vi "Version_4.9_8_on-chip_valves_for25ulSyringe_withModfied_Plunging.vi"() -> ()   [LabVIEW 2020] (continued)
                                n4611 = local read "VISA Refnum in\nfor Pump"() -> (w5031:refnum<visa-resource-name>)
                                n4612 = local read "Initial Plunger Position"() -> (w5030:dbl)
                                n4613 = local read "Volume of Syringe"() -> (w5028:dbl)
                                n4614 = while {
                                tunnel: w5030 -> [w5038]
                                tunnel: w5031 -> [w5037]
                                tunnel: w5029 -> [w5036]
                                tunnel: w5028 -> [w5035]
                                stop <- w5033 stop-if-true
                                n4615 = stacked-sequence {
                                tunnel: w5038 -> [w5045 _]
                                tunnel: w5037 -> [w5044 w5065]
                                tunnel: w5036 -> [w5043 _]
                                tunnel: w5035 -> [w5042 _]
                                tunnel: [_ w5063] -> w5033
                                frame #0 {
                                n4616 = call "AbsolutePlungerPosition (SubVI).vi"("VISA Refnum in"=w5044) -> ("Plunger Position"=w5041:i32)  [unwired: 10 in]
                                n4617 = case shown="\"Standard Pumping\", Default" w5043 {
                                tunnel: w5045 -> [w5050 w5059]
                                tunnel: w5041 -> [w5051 w5058]
                                tunnel: [w5049 w5056] -> w5040
                                tunnel: w5042 -> [w5048 w5057]
                                frame "Standard Pumping", Default {
                                n4618 = Subtract(x=w5050, y=w5051) -> (x-y=w5047:dbl)
                                n4619 = Absolute Value(x=w5047) -> (abs(x)=w5046:dbl)
                                n4620 = Multiply(x=w5046, y=w5048) -> (x*y=w5053:dbl)
                                n4621 = Divide(x=w5053, y=3000.0) -> (x/y=w5049:dbl)
                                }
                                frame "High Resolution Pumping" {
                                n4622 = Subtract(x=w5059, y=w5058) -> (x-y=w5055:dbl)
                                n4623 = Absolute Value(x=w5055) -> (abs(x)=w5054:dbl)
                                n4624 = Multiply(x=w5054, y=w5057) -> (x*y=w5061:dbl)
                                n4625 = Divide(x=w5061, y=24000.0) -> (x/y=w5056:dbl)
                                }
                                }
                                n4626 = local write "Volume being Injected \nin this process"(w5040) -> ()
                                }
                                frame #1 {
                                n4627 = local read "Stopper that ends \nthe main loops"() -> (w5062:bool)
                                n4628 = call "LSPOneStatus (SubVI).vi"("VISA Refnum in"=w5065) -> ("read buffer"=w5067:string)  [unwired: 10 in]
                                n4629 = call <vilib>:"Trim Whitespace.vi"("string"=w5067) -> ("trimmed string"=w5066:string)  [unwired: 1 in]
                                n4630 = Equal?(x=w5066, y="/0`\u0003") -> (x = y?=w5064:bool)
                                n4631 = Or(x=w5064, y=w5062) -> (x .or. y?=w5063:bool)
                                }
                                }
                                n4632 = Wait (ms)(milliseconds to wait=u32 100) -> ()  [unwired: 1 out]
                                n4633 = local read "Stopper that ends \nthe main loops"() -> (w5032:bool)
                                n4634 = case shown="True" w5032 {
                                frame False {
                                }
                                frame True {
                                n4635 = local read "VISA Refnum in\nfor Pump"() -> (w5039:refnum<visa-resource-name>)
                                n4636 = call "HardStopCurrentProcess (SubVI).vi"("VISA Refnum in"=w5039) -> ()  [unwired: 11 in]
                                }
                                }
                                }
                              }
                              frame #9 {
                                n4637 = local write "Pause Data Collection"(TRUE ("Pause Data Collection")) -> ()
                                n4638 = Wait (ms)(milliseconds to wait=u32 500) -> ()  [unwired: 1 out]
                              }
                              frame #10 {
                                n4639 = local write "Volume being Injected \nin this process"(0.0 ("Volume being Injected \nin this process")) -> ()
                                n4640 = local write "Start the Process"(FALSE ("Start the Process")) -> ()
                              }
                            }
                          }
                          frame #16 {
                            # "Clean the tubing with Sample"
                            n4641 = local read "N-S"() -> (w5073:i32)
                            n4642 = for {
                              N: w5073 -> [_]
                              n4643 = stacked-sequence {
                                frame #0 {
                                n4644 = local read "VISA Refnum in\nfor Pump"() -> (w5076:refnum<visa-resource-name>)
                                n4645 = local read "Port for \nSample"() -> (w5075:string)
                                n4646 = call "PortChanger (SubVI).vi"("Port Number"=w5075, "VISA Refnum in"=w5076) -> ()  [unwired: 10 in]
                                }
                                frame #1 {
                                n4647 = local read "VISA Refnum in\nfor Pump"() -> (w5077:refnum<visa-resource-name>)
                                n4648 = call "ProcessCompletionWaiter (SubVI).vi"("VISA Refnum in"=w5077) -> ()  [unwired: 11 in]
                                }
                                frame #2 {
                                n4649 = local read "VISA Refnum in\nfor Pump"() -> (w5082:refnum<visa-resource-name>)
                                n4650 = local read "Sample PickUp \nFlow Rate (ul/min)"() -> (w5079:dbl)
                                n4651 = local read "V-S"() -> (w5078:dbl)
                                n4652 = local read "Volume of Syringe"() -> (w5080:dbl)
                                n4653 = call "RPickUp(SubVI).vi"("Volume to be picked up"=w5078, "Volume of Syringe"=w5080, "Resolution of PickUP"=T2."Standard Pumping", "PickUp Flow Rate (ul/min)"=w5079, "VISA Refnum in"=w5082) -> ()  [unwired: 6 in, 1 out]
                                }
                                frame #3 {
                                n4654 = local read "Stopper that ends \nthe main loops"() -> (w5083:bool)
                                n4655 = local read "VISA Refnum in\nfor Pump"() -> (w5084:refnum<visa-resource-name>)
                                n4656 = case shown="True" w5083 {
                                frame False {
                                }
                                frame True {
                                n4657 = local read "VISA Refnum in\nfor Pump"() -> (w5085:refnum<visa-resource-name>)
                                n4658 = call "HardStopCurrentProcess (SubVI).vi"("VISA Refnum in"=w5085) -> ()  [unwired: 11 in]
                                }
                                }
                                n4659 = call "ProcessCompletionWaiter (SubVI).vi"("VISA Refnum in"=w5084) -> ()  [unwired: 11 in]
                                }
                                frame #4 {
                                n4660 = local read "VISA Refnum in\nfor Pump"() -> (w5087:refnum<visa-resource-name>)
                                n4661 = call "PortChanger (SubVI).vi"("Port Number"="1", "VISA Refnum in"=w5087) -> ()  [unwired: 10 in]
                                }
                                frame #5 {
                                n4662 = local read "Stopper that ends \nthe main loops"() -> (w5088:bool)
                                n4663 = local read "VISA Refnum in\nfor Pump"() -> (w5089:refnum<visa-resource-name>)
                                n4664 = case shown="True" w5088 {
                                frame False {
                                }
                                frame True {
                                n4665 = local read "VISA Refnum in\nfor Pump"() -> (w5090:refnum<visa-resource-name>)
                                n4666 = call "HardStopCurrentProcess (SubVI).vi"("VISA Refnum in"=w5090) -> ()  [unwired: 11 in]
                                }
                                }
                                n4667 = call "ProcessCompletionWaiter (SubVI).vi"("VISA Refnum in"=w5089) -> ()  [unwired: 11 in]
                                }
                                frame #6 {
                                n4668 = local read "VISA Refnum in\nfor Pump"() -> (w5095:refnum<visa-resource-name>)
                                n4669 = local read "Volume of Syringe"() -> (w5092:dbl)
                                n4670 = call "GoToAbsolutePosition(SubVI).vi"("Absolute Volume Position in Syringe (in ul)"=0.0 ("Volume to be picked up"), "Volume of Syringe"=w5092, "Resolution of Pumping"=T2."Standard Pumping" ("Resolution of PickUP"), "Flow Rate (ul/min)"=150.0 ("PickUp Flow Rate (ul/min)"), "VISA Refnum in"=w5095) -> ()  [unwired: 6 in, 1 out]
                                }
                                frame #7 {
                                n4671 = local read "Stopper that ends \nthe main loops"() -> (w5096:bool)
                                n4672 = local read "VISA Refnum in\nfor Pump"() -> (w5097:refnum<visa-resource-name>)
                                n4673 = case shown="True" w5096 {
                                frame False {
                                }
                                frame True {
                                n4674 = local read "VISA Refnum in\nfor Pump"() -> (w5098:refnum<visa-resource-name>)
                                n4675 = call "HardStopCurrentProcess (SubVI).vi"("VISA Refnum in"=w5098) -> ()  [unwired: 11 in]
                                }
                                }
                                n4676 = call "ProcessCompletionWaiter (SubVI).vi"("VISA Refnum in"=w5097) -> ()  [unwired: 11 in]
                                }
                              }
                              n4677 = local write "Pause Data Collection"(TRUE ("Pause Data Collection")) -> ()
                            }
                          }
                        }
                      }
                      frame #1 {
                        # "Pump Sample into Column-1"
                        n4678 = stacked-sequence {
                          frame #0 {
                            # "Switch to Port-3"
                            # "Port-3 of pump is connected to Sample"
                            n4679 = local read "VISA Refnum in\nfor Pump"() -> (w5103:refnum<visa-resource-name>)
                            n4680 = local read "Port for \nSample"() -> (w5102:string)
                            n4681 = call "PortChanger (SubVI).vi"("Port Number"=w5102, "VISA Refnum in"=w5103) -> ()  [unwired: 10 in]
                          }
                          frame #1 {
                            n4682 = local read "VISA Refnum in\nfor Pump"() -> (w5104:refnum<visa-resource-name>)
                            n4683 = call "ProcessCompletionWaiter (SubVI).vi"("VISA Refnum in"=w5104) -> ()  [unwired: 11 in]
                          }
                          frame #2 {
                            n4684 = local write "Valve V1 Open"(TRUE ("Valve V1 Open")) -> ()
                            n4685 = local write "Valve V2 Open"(TRUE ("Valve V2 Open")) -> ()
                            n4686 = local write "Valve V3 Open"(FALSE ("Valve V3 Open")) -> ()
                            n4687 = local write "Valve V4 Open"(FALSE ("Valve V4 Open")) -> ()
                            n4688 = local write "External Valve \nOpen"(TRUE ("External Valve \nOpen")) -> ()
                            n4689 = local write "Valve V5 Open"(FALSE ("Valve V5 Open")) -> ()
                            n4690 = local write "Valve V8 Open"(FALSE ("Valve V8 Open")) -> ()
                            n4691 = local write "Valve V6 Open"(FALSE ("Valve V6 Open")) -> ()
                            n4692 = local write "Valve V7 Open"(FALSE ("Valve V7 Open")) -> ()
                          }
                          frame #3 {
                            n4693 = local read "Apparent Volume\nof Syringe"() -> (w5114:dbl)
                            n4694 = local read "Sample Volume \nto be Pumped"() -> (w5117:dbl)
                            n4695 = Quotient & Remainder(x=w5117, y=w5114) -> (x-y*floor(x/y)=w5115:dbl, floor(x/y)=w5116:dbl)
                            n4696 = for {
                              N: w5116 -> [_]
                              n4697 = stacked-sequence {
                                frame #0 {
                                n4698 = local read "Sample PickUp \nFlow Rate (ul/min)"() -> (w5120:dbl)
                                n4699 = local read "Sample Pumping\nResolution"() -> (w5119:T2)
                                n4700 = local read "VISA Refnum in\nfor Pump"() -> (w5122:refnum<visa-resource-name>)
                                n4701 = local read "Apparent Volume\nof Syringe"() -> (w5118:dbl)
                                n4702 = local read "Volume of Syringe"() -> (w5121:dbl)
                                n4703 = call "RPickUp(SubVI).vi"("Volume to be picked up"=w5118, "Volume of Syringe"=w5121, "Resolution of PickUP"=w5119, "PickUp Flow Rate (ul/min)"=w5120, "VISA Refnum in"=w5122) -> ()  [unwired: 6 in, 1 out]
                                }
                                frame #1 {
                                n4704 = local read "Stopper that ends \nthe main loops"() -> (w5123:bool)
                                n4705 = local read "VISA Refnum in\nfor Pump"() -> (w5124:refnum<visa-resource-name>)
                                n4706 = case shown="True" w5123 {
                                frame False {
                                }
                                frame True {
                                n4707 = local read "VISA Refnum in\nfor Pump"() -> (w5125:refnum<visa-resource-name>)
                                n4708 = call "HardStopCurrentProcess (SubVI).vi"("VISA Refnum in"=w5125) -> ()  [unwired: 11 in]
                                }
                                }
                                n4709 = call "ProcessCompletionWaiter (SubVI).vi"("VISA Refnum in"=w5124) -> ()  [unwired: 11 in]
                                }
                                frame #2 {
                                # "Reads the initial Plunger Position for computing the volume dispensed"
                                n4710 = local read "VISA Refnum in\nfor Pump"() -> (w5127:refnum<visa-resource-name>)
                                n4711 = call "AbsolutePlungerPosition (SubVI).vi"("VISA Refnum in"=w5127) -> ("Plunger Position"=w5126:i32)  [unwired: 10 in]
                                n4712 = local write "Initial Plunger Position"(w5126) -> ()
                                }
                                frame #3 {
                                # "Switch to Port-2"
                                # "Port-2 of the pump is conncted to column-1 of chip"
                                n4713 = local read "VISA Refnum in\nfor Pump"() -> (w5129:refnum<visa-resource-name>)
                                n4714 = call "PortChanger (SubVI).vi"("Port Number"="2", "VISA Refnum in"=w5129) -> ()  [unwired: 10 in]
                                }
                                frame #4 {
                                n4715 = local read "Stopper that ends \nthe main loops"() -> (w5130:bool)
                                n4716 = local read "VISA Refnum in\nfor Pump"() -> (w5131:refnum<visa-resource-name>)
                                n4717 = case shown="True" w5130 {
                                frame False {
                                }
                                frame True {
                                n4718 = local read "VISA Refnum in\nfor Pump"() -> (w5132:refnum<visa-resource-name>)
                                n4719 = call "HardStopCurrentProcess (SubVI).vi"("VISA Refnum in"=w5132) -> ()  [unwired: 11 in]
                                }
                                }
                                n4720 = call "ProcessCompletionWaiter (SubVI).vi"("VISA Refnum in"=w5131) -> ()  [unwired: 11 in]
                                }
                                frame #5 {
                                # "Keeps the AMF valve after column-1 open and valve after column-2 closed"
                                n4721 = local read "Sample Dispense\nFlow Rate (ul/min)"() -> (w5136:dbl)
                                n4722 = local read "Sample Pumping\nResolution"() -> (w5135:T2)
                                n4723 = local read "VISA Refnum in\nfor Pump"() -> (w5138:refnum<visa-resource-name>)
                                n4724 = local write "Pause Data Collection"(FALSE ("Pause Data Collection")) -> ()
                                n4725 = local read "Volume of Syringe"() -> (w5137:dbl)
                                n4726 = call "GoToAbsolutePosition(SubVI).vi"("Absolute Volume Position in Syringe (in ul)"=0.0 ("Volume to be Dispensed"), "Volume of Syringe"=w5137, "Resolution of Pumping"=w5135, "Flow Rate (ul/min)"=w5136, "VISA Refnum in"=w5138) -> ()  [unwired: 6 in, 1 out]
                                }
                                frame #6 {
                                n4727 = local read "Sample Pumping\nResolution"() -> (w5140:T2)
                                n4728 = local read "VISA Refnum in\nfor Pump"() -> (w5142:refnum<visa-resource-name>)
                                n4729 = local read "Initial Plunger Position"() -> (w5141:dbl)
                                n4730 = local read "Volume of Syringe"() -> (w5139:dbl)
                                n4731 = while {
                                tunnel: w5141 -> [w5149]
                                tunnel: w5142 -> [w5148]
                                tunnel: w5140 -> [w5147]
                                tunnel: w5139 -> [w5146]
                                stop <- w5144 stop-if-true
                                n4732 = stacked-sequence {
                                tunnel: w5149 -> [w5156 _]
                                tunnel: w5148 -> [w5155 w5176]
                                tunnel: w5147 -> [w5154 _]
                                tunnel: w5146 -> [w5153 _]
                                tunnel: [_ w5174] -> w5144
                                frame #0 {
                                n4733 = call "AbsolutePlungerPosition (SubVI).vi"("VISA Refnum in"=w5155) -> ("Plunger Position"=w5152:i32)  [unwired: 10 in]
                                n4734 = case shown="\"Standard Pumping\", Default" w5154 {
                                tunnel: w5156 -> [w5161 w5170]
                                tunnel: w5152 -> [w5162 w5169]
                                tunnel: [w5160 w5167] -> w5151
                                tunnel: w5153 -> [w5159 w5168]
                                frame "Standard Pumping", Default {
                                n4735 = Subtract(x=w5161, y=w5162) -> (x-y=w5158:dbl)
                                n4736 = Absolute Value(x=w5158) -> (abs(x)=w5157:dbl)
                                n4737 = Multiply(x=w5157, y=w5159) -> (x*y=w5164:dbl)
                                n4738 = Divide(x=w5164, y=3000.0) -> (x/y=w5160:dbl)
                                }
                                frame "High Resolution Pumping" {
                                n4739 = Subtract(x=w5170, y=w5169) -> (x-y=w5166:dbl)
                                n4740 = Absolute Value(x=w5166) -> (abs(x)=w5165:dbl)
                                n4741 = Multiply(x=w5165, y=w5168) -> (x*y=w5172:dbl)
                                n4742 = Divide(x=w5172, y=24000.0) -> (x/y=w5167:dbl)
                                }
                                }
                                n4743 = local write "Volume being Injected \nin this process"(w5151) -> ()
                                }
                                frame #1 {
                                n4744 = call "LSPOneStatus (SubVI).vi"("VISA Refnum in"=w5176) -> ("read buffer"=w5178:string)  [unwired: 10 in]
                                n4745 = call <vilib>:"Trim Whitespace.vi"("string"=w5178) -> ("trimmed string"=w5177:string)  [unwired: 1 in]
                                n4746 = local read "Stopper that ends \nthe main loops"() -> (w5173:bool)
                                n4747 = Equal?(x=w5177, y="/0`\u0003") -> (x = y?=w5175:bool)
                                n4748 = Or(x=w5175, y=w5173) -> (x .or. y?=w5174:bool)
                                }
                                }
                                n4749 = Wait (ms)(milliseconds to wait=u32 100) -> ()  [unwired: 1 out]
                                n4750 = local read "Stopper that ends \nthe main loops"() -> (w5143:bool)
                                n4751 = case shown="True" w5143 {
                                frame False {
                                }
                                frame True {
                                n4752 = local read "VISA Refnum in\nfor Pump"() -> (w5150:refnum<visa-resource-name>)
                                n4753 = call "HardStopCurrentProcess (SubVI).vi"("VISA Refnum in"=w5150) -> ()  [unwired: 11 in]
                                }
                                }
                                }
                                }
                                frame #7 {
                                # "Chnage the pump port back to Sample"
                                n4754 = local read "VISA Refnum in\nfor Pump"() -> (w5181:refnum<visa-resource-name>)
                                n4755 = local read "Port for \nSample"() -> (w5180:string)
                                n4756 = local write "Pause Data Collection"(TRUE ("Pause Data Collection")) -> ()
                                n4757 = Wait (ms)(milliseconds to wait=u32 500) -> ()  [unwired: 1 out]
                                n4758 = call "PortChanger (SubVI).vi"("Port Number"=w5180, "VISA Refnum in"=w5181) -> ()  [unwired: 10 in]
                                }
                                frame #8 {
                                n4759 = local read "VISA Refnum in\nfor Pump"() -> (w5184:refnum<visa-resource-name>)
                                n4760 = local write "Volume being Injected \nin this process"(0.0 ("Volume being Injected \nin this process")) -> ()
                                n4761 = call "ProcessCompletionWaiter (SubVI).vi"("VISA Refnum in"=w5184) -> ()  [unwired: 11 in]
                                }
                              }
                            }
                            n4762 = local write "Reminder of the \nVolume to be \nPumped"(w5115) -> ()
                          }
                          frame #4 {
                            n4763 = stacked-sequence {
                              frame #0 {
                                n4764 = local read "Sample PickUp \nFlow Rate (ul/min)"() -> (w5188:dbl)
                                n4765 = local read "Sample Pumping\nResolution"() -> (w5187:T2)
                                n4766 = local read "VISA Refnum in\nfor Pump"() -> (w5190:refnum<visa-resource-name>)
                                n4767 = local read "Reminder of the \nVolume to be \nPumped"() -> (w5186:dbl)
                                n4768 = local read "Volume of Syringe"() -> (w5189:dbl)
                                n4769 = call "RPickUp(SubVI).vi"("Volume to be picked up"=w5186, "Volume of Syringe"=w5189, "Resolution of PickUP"=w5187, "PickUp Flow Rate (ul/min)"=w5188, "VISA Refnum in"=w5190) -> ()  [unwired: 6 in, 1 out]
                              }
                              frame #1 {
                                n4770 = local read "Stopper that ends \nthe main loops"() -> (w5191:bool)
                                n4771 = local read "VISA Refnum in\nfor Pump"() -> (w5192:refnum<visa-resource-name>)
                                n4772 = case shown="True" w5191 {
                                frame False {
                                }
                                frame True {
                                n4773 = local read "VISA Refnum in\nfor Pump"() -> (w5193:refnum<visa-resource-name>)
                                n4774 = call "HardStopCurrentProcess (SubVI).vi"("VISA Refnum in"=w5193) -> ()  [unwired: 11 in]
                                }
                                }
                                n4775 = call "ProcessCompletionWaiter (SubVI).vi"("VISA Refnum in"=w5192) -> ()  [unwired: 11 in]
                              }
                              frame #2 {
                                # "Reads the initial Plunger Position for computing the volume dispensed"
                                n4776 = local read "VISA Refnum in\nfor Pump"() -> (w5195:refnum<visa-resource-name>)
                                n4777 = call "AbsolutePlungerPosition (SubVI).vi"("VISA Refnum in"=w5195) -> ("Plunger Position"=w5194:i32)  [unwired: 10 in]
                                n4778 = local write "Initial Plunger Position"(w5194) -> ()
                              }
                              frame #3 {
                                # "Switch to Port-2"
                                # "Port-2 of the pump is conncted to column-1 of chip"
                                n4779 = local read "VISA Refnum in\nfor Pump"() -> (w5197:refnum<visa-resource-name>)
                                n4780 = call "PortChanger (SubVI).vi"("Port Number"="2", "VISA Refnum in"=w5197) -> ()  [unwired: 10 in]
                              }
                              frame #4 {
                                n4781 = local read "Stopper that ends \nthe main loops"() -> (w5198:bool)
                                n4782 = local read "VISA Refnum in\nfor Pump"() -> (w5199:refnum<visa-resource-name>)
                                n4783 = case shown="True" w5198 {
                                frame False {
                                }
                                frame True {
                                n4784 = local read "VISA Refnum in\nfor Pump"() -> (w5200:refnum<visa-resource-name>)
                                n4785 = call "HardStopCurrentProcess (SubVI).vi"("VISA Refnum in"=w5200) -> ()  [unwired: 11 in]
                                }
                                }
                                n4786 = call "ProcessCompletionWaiter (SubVI).vi"("VISA Refnum in"=w5199) -> ()  [unwired: 11 in]
                              }
                              frame #5 {
                                # "Keeps the AMF valve after column-1 open and valve after column-2 closed"
                                n4787 = local read "Sample Dispense\nFlow Rate (ul/min)"() -> (w5204:dbl)
                                n4788 = local read "Sample Pumping\nResolution"() -> (w5203:T2)
                                n4789 = local read "VISA Refnum in\nfor Pump"() -> (w5206:refnum<visa-resource-name>)
                                n4790 = local write "Pause Data Collection"(FALSE ("Pause Data Collection")) -> ()
                                n4791 = local read "Volume of Syringe"() -> (w5205:dbl)
                                n4792 = call "GoToAbsolutePosition(SubVI).vi"("Absolute Volume Position in Syringe (in ul)"=0.0 ("Volume to be Dispensed"), "Volume of Syringe"=w5205, "Resolution of Pumping"=w5203, "Flow Rate (ul/min)"=w5204, "VISA Refnum in"=w5206) -> ()  [unwired: 6 in, 1 out]
                              }
                              frame #6 {
                                n4793 = local read "Sample Pumping\nResolution"() -> (w5208:T2)
                                n4794 = local read "VISA Refnum in\nfor Pump"() -> (w5210:refnum<visa-resource-name>)
                                n4795 = local read "Initial Plunger Position"() -> (w5209:dbl)
                                n4796 = local read "Volume of Syringe"() -> (w5207:dbl)
                                n4797 = while {
                                tunnel: w5209 -> [w5217]
                                tunnel: w5210 -> [w5216]
                                tunnel: w5208 -> [w5215]
                                tunnel: w5207 -> [w5214]
                                stop <- w5212 stop-if-true
                                n4798 = stacked-sequence {
                                tunnel: w5217 -> [w5224 _]
                                tunnel: w5216 -> [w5223 w5244]
                                tunnel: w5215 -> [w5222 _]
                                tunnel: w5214 -> [w5221 _]
                                tunnel: [_ w5242] -> w5212
                                frame #0 {
                                n4799 = call "AbsolutePlungerPosition (SubVI).vi"("VISA Refnum in"=w5223) -> ("Plunger Position"=w5220:i32)  [unwired: 10 in]
                                n4800 = case shown="\"Standard Pumping\", Default" w5222 {
                                tunnel: w5224 -> [w5229 w5238]
                                tunnel: w5220 -> [w5230 w5237]
                                tunnel: [w5228 w5235] -> w5219
                                tunnel: w5221 -> [w5227 w5236]
                                frame "Standard Pumping", Default {
                                n4801 = Subtract(x=w5229, y=w5230) -> (x-y=w5226:dbl)
                                n4802 = Absolute Value(x=w5226) -> (abs(x)=w5225:dbl)
                                n4803 = Multiply(x=w5225, y=w5227) -> (x*y=w5232:dbl)
                                n4804 = Divide(x=w5232, y=3000.0) -> (x/y=w5228:dbl)
                                }
                                frame "High Resolution Pumping" {
                                n4805 = Subtract(x=w5238, y=w5237) -> (x-y=w5234:dbl)
                                n4806 = Absolute Value(x=w5234) -> (abs(x)=w5233:dbl)
                                n4807 = Multiply(x=w5233, y=w5236) -> (x*y=w5240:dbl)
                                n4808 = Divide(x=w5240, y=24000.0) -> (x/y=w5235:dbl)
                                }
                                }
                                n4809 = local write "Volume being Injected \nin this process"(w5219) -> ()
                                }
                                frame #1 {
                                n4810 = call "LSPOneStatus (SubVI).vi"("VISA Refnum in"=w5244) -> ("read buffer"=w5246:string)  [unwired: 10 in]
                                n4811 = call <vilib>:"Trim Whitespace.vi"("string"=w5246) -> ("trimmed string"=w5245:string)  [unwired: 1 in]
                                n4812 = local read "Stopper that ends \nthe main loops"() -> (w5241:bool)
                                n4813 = Equal?(x=w5245, y="/0`\u0003") -> (x = y?=w5243:bool)
                                n4814 = Or(x=w5243, y=w5241) -> (x .or. y?=w5242:bool)
                                }
                                }
                                n4815 = Wait (ms)(milliseconds to wait=u32 100) -> ()  [unwired: 1 out]
                                n4816 = local read "Stopper that ends \nthe main loops"() -> (w5211:bool)
                                n4817 = case shown="True" w5211 {
                                frame False {
                                }
                                frame True {
                                n4818 = local read "VISA Refnum in\nfor Pump"() -> (w5218:refnum<visa-resource-name>)
                                n4819 = call "HardStopCurrentProcess (SubVI).vi"("VISA Refnum in"=w5218) -> ()  [unwired: 11 in]
                                }
                                }
                                }
                              }
                              frame #7 {
                                n4820 = local write "Pause Data Collection"(TRUE ("Pause Data Collection")) -> ()
                                n4821 = Wait (ms)(milliseconds to wait=u32 500) -> ()  [unwired: 1 out]
                              }
                              frame #8 {
                                n4822 = local write "Volume being Injected \nin this process"(0.0 ("Volume being Injected \nin this process")) -> ()
                              }
                            }
                          }
                        }
                        n4823 = local write "Equilibriating \nColumn-2"(FALSE ("Equilibriating \nColumn-2")) -> ()
                        n4824 = local write "Affinity On"(TRUE ("Affinity On")) -> ()
                        n4825 = local write "Sample pumping \ninto Column-1"(TRUE ("Sample pumping \ninto Column-1")) -> ()
                      }
                      frame #2 {
                        # "Wash Column-1 with Buffer-A2"
                        n4826 = local write "Sample pumping \ninto Column-1"(FALSE ("Sample pumping \ninto Column-1")) -> ()
                        n4827 = stacked-sequence {
                          frame #0 {
                            # "Switch to Port-4/6"
                            # "Port-4/6 of pump is connected to Buffer-A2"
                            n4828 = local read "VISA Refnum in\nfor Pump"() -> (w5254:refnum<visa-resource-name>)
                            n4829 = local read "Port for \nA2-Wash"() -> (w5253:string)
                            n4830 = call "PortChanger (SubVI).vi"("Port Number"=w5253, "VISA Refnum in"=w5254) -> ()  [unwired: 10 in]
                          }
                          frame #1 {
                            n4831 = local read "VISA Refnum in\nfor Pump"() -> (w5255:refnum<visa-resource-name>)
                            n4832 = call "ProcessCompletionWaiter (SubVI).vi"("VISA Refnum in"=w5255) -> ()  [unwired: 11 in]
                          }
                          frame #2 {
                            n4833 = local write "Valve V3 Open"(FALSE ("Valve V3 Open")) -> ()
                            n4834 = local write "Valve V4 Open"(FALSE ("Valve V4 Open")) -> ()
                            n4835 = local write "Valve V1 Open"(TRUE ("Valve V1 Open")) -> ()
                            n4836 = local write "Valve V2 Open"(TRUE ("Valve V2 Open")) -> ()
                            n4837 = local write "External Valve \nOpen"(TRUE ("Elution of Column-2")) -> ()
                            n4838 = local write "Valve V8 Open"(FALSE ("Valve V8 Open")) -> ()
                            n4839 = local write "Valve V5 Open"(FALSE ("Valve V5 Open")) -> ()
                            n4840 = local write "Valve V6 Open"(FALSE ("Valve V6 Open")) -> ()
                            n4841 = local write "Valve V7 Open"(FALSE ("Valve V7 Open")) -> ()
                          }
                          frame #3 {
                            n4842 = local read "Buffer-A2 Volume \nto be Pumped"() -> (w5268:dbl)
                            n4843 = local read "Apparent Volume\nof Syringe"() -> (w5265:dbl)
                            n4844 = Quotient & Remainder(x=w5268, y=w5265) -> (x-y*floor(x/y)=w5266:dbl, floor(x/y)=w5267:dbl)
                            n4845 = for {
                              N: w5267 -> [_]
                              n4846 = stacked-sequence {
                                frame #0 {
                                n4847 = local read "Buffer-A2 PickUp \nFlow Rate (ul/min)"() -> (w5271:dbl)
                                n4848 = local read "Buffer-A2 Pumping\nResolution"() -> (w5270:T2)
                                n4849 = local read "VISA Refnum in\nfor Pump"() -> (w5273:refnum<visa-resource-name>)
                                n4850 = local read "Apparent Volume\nof Syringe"() -> (w5269:dbl)
                                n4851 = local read "Volume of Syringe"() -> (w5272:dbl)
                                n4852 = call "RPickUp(SubVI).vi"("Volume to be picked up"=w5269, "Volume of Syringe"=w5272, "Resolution of PickUP"=w5270, "PickUp Flow Rate (ul/min)"=w5271, "VISA Refnum in"=w5273) -> ()  [unwired: 6 in, 1 out]
                                }
                                frame #1 {
                                n4853 = local read "Stopper that ends \nthe main loops"() -> (w5274:bool)
                                n4854 = local read "VISA Refnum in\nfor Pump"() -> (w5275:refnum<visa-resource-name>)
                                n4855 = case shown="True" w5274 {
                                frame False {
                                }
                                frame True {
                                n4856 = local read "VISA Refnum in\nfor Pump"() -> (w5276:refnum<visa-resource-name>)
                                n4857 = call "HardStopCurrentProcess (SubVI).vi"("VISA Refnum in"=w5276) -> ()  [unwired: 11 in]
                                }
                                }
                                n4858 = call "ProcessCompletionWaiter (SubVI).vi"("VISA Refnum in"=w5275) -> ()  [unwired: 11 in]
                                }
                                frame #2 {
                                # "Reads the initial Plunger Position for computing the volume dispensed"
                                n4859 = local read "VISA Refnum in\nfor Pump"() -> (w5278:refnum<visa-resource-name>)
                                n4860 = call "AbsolutePlungerPosition (SubVI).vi"("VISA Refnum in"=w5278) -> ("Plunger Position"=w5277:i32)  [unwired: 10 in]
                                n4861 = local write "Initial Plunger Position"(w5277) -> ()
                                }
                                frame #3 {
                                # "Switch to Port-2"
                                # "Port-2 of the pump is conncted to column-1 of chip"
                                n4862 = local read "VISA Refnum in\nfor Pump"() -> (w5280:refnum<visa-resource-name>)
                                n4863 = call "PortChanger (SubVI).vi"("Port Number"="2", "VISA Refnum in"=w5280) -> ()  [unwired: 10 in]
                                }
                                frame #4 {
                                n4864 = local read "Stopper that ends \nthe main loops"() -> (w5281:bool)
                                n4865 = local read "VISA Refnum in\nfor Pump"() -> (w5282:refnum<visa-resource-name>)
                                n4866 = case shown="True" w5281 {
                                frame False {
                                }
                                frame True {
                                n4867 = local read "VISA Refnum in\nfor Pump"() -> (w5283:refnum<visa-resource-name>)
                                n4868 = call "HardStopCurrentProcess (SubVI).vi"("VISA Refnum in"=w5283) -> ()  [unwired: 11 in]
                                }
                                }
                                n4869 = call "ProcessCompletionWaiter (SubVI).vi"("VISA Refnum in"=w5282) -> ()  [unwired: 11 in]
                                }
                                frame #5 {
                                # "Keeps the AMF valve after column-1 open and valve after column-2 closed"
                                n4870 = local read "Buffer-A2 Dispense\nFlow Rate (ul/min)"() -> (w5287:dbl)
                                n4871 = local read "Buffer-A2 Pumping\nResolution"() -> (w5286:T2)
                                n4872 = local read "VISA Refnum in\nfor Pump"() -> (w5289:refnum<visa-resource-name>)
                                n4873 = local write "Pause Data Collection"(FALSE ("Pause Data Collection")) -> ()
                                n4874 = local read "Volume of Syringe"() -> (w5288:dbl)
                                n4875 = call "GoToAbsolutePosition(SubVI).vi"("Absolute Volume Position in Syringe (in ul)"=0.0 ("Volume to be Dispensed"), "Volume of Syringe"=w5288, "Resolution of Pumping"=w5286, "Flow Rate (ul/min)"=w5287, "VISA Refnum in"=w5289) -> ()  [unwired: 6 in, 1 out]
                                }
                                frame #6 {
                                n4876 = local read "Buffer-A2 Pumping\nResolution"() -> (w5291:T2)
                                n4877 = local read "VISA Refnum in\nfor Pump"() -> (w5293:refnum<visa-resource-name>)
                                n4878 = local read "Initial Plunger Position"() -> (w5292:dbl)
                                n4879 = local read "Volume of Syringe"() -> (w5290:dbl)
                                n4880 = while {
                                tunnel: w5292 -> [w5300]
                                tunnel: w5293 -> [w5299]
                                tunnel: w5291 -> [w5298]
                                tunnel: w5290 -> [w5297]
                                stop <- w5295 stop-if-true
                                n4881 = stacked-sequence {
                                tunnel: w5300 -> [w5307 _]
                                tunnel: w5299 -> [w5306 w5327]
                                tunnel: w5298 -> [w5305 _]
                                tunnel: w5297 -> [w5304 _]
                                tunnel: [_ w5325] -> w5295
                                frame #0 {
                                n4882 = call "AbsolutePlungerPosition (SubVI).vi"("VISA Refnum in"=w5306) -> ("Plunger Position"=w5303:i32)  [unwired: 10 in]
                                n4883 = case shown="\"Standard Pumping\", Default" w5305 {
                                tunnel: w5307 -> [w5312 w5321]
                                tunnel: w5303 -> [w5313 w5320]
                                tunnel: [w5311 w5318] -> w5302
                                tunnel: w5304 -> [w5310 w5319]
                                frame "Standard Pumping", Default {
                                n4884 = Subtract(x=w5312, y=w5313) -> (x-y=w5309:dbl)
                                n4885 = Absolute Value(x=w5309) -> (abs(x)=w5308:dbl)
                                n4886 = Multiply(x=w5308, y=w5310) -> (x*y=w5315:dbl)
                                n4887 = Divide(x=w5315, y=3000.0) -> (x/y=w5311:dbl)
                                }
                                frame "High Resolution Pumping" {
                                n4888 = Subtract(x=w5321, y=w5320) -> (x-y=w5317:dbl)
                                n4889 = Absolute Value(x=w5317) -> (abs(x)=w5316:dbl)
                                n4890 = Multiply(x=w5316, y=w5319) -> (x*y=w5323:dbl)
                                n4891 = Divide(x=w5323, y=24000.0) -> (x/y=w5318:dbl)
                                }
                                }
                                n4892 = local write "Volume being Injected \nin this process"(w5302) -> ()
                                }
                                frame #1 {
                                n4893 = call "LSPOneStatus (SubVI).vi"("VISA Refnum in"=w5327) -> ("read buffer"=w5329:string)  [unwired: 10 in]
                                n4894 = call <vilib>:"Trim Whitespace.vi"("string"=w5329) -> ("trimmed string"=w5328:string)  [unwired: 1 in]
                                n4895 = local read "Stopper that ends \nthe main loops"() -> (w5324:bool)
                                n4896 = Equal?(x=w5328, y="/0`\u0003") -> (x = y?=w5326:bool)
                                n4897 = Or(x=w5326, y=w5324) -> (x .or. y?=w5325:bool)
                                }
                                }
                                n4898 = Wait (ms)(milliseconds to wait=u32 100) -> ()  [unwired: 1 out]
                                n4899 = local read "Stopper that ends \nthe main loops"() -> (w5294:bool)
                                n4900 = case shown="True" w5294 {
                                frame False {
                                }
                                frame True {
                                n4901 = local read "VISA Refnum in\nfor Pump"() -> (w5301:refnum<visa-resource-name>)
                                n4902 = call "HardStopCurrentProcess (SubVI).vi"("VISA Refnum in"=w5301) -> ()  [unwired: 11 in]
                                }
                                }
                                }
                                }
                                frame #7 {
                                # "Change the port back to Buffer-A2"
                                n4903 = local read "VISA Refnum in\nfor Pump"() -> (w5332:refnum<visa-resource-name>)
                                n4904 = local read "Port for \nA2-Wash"() -> (w5331:string)
                                n4905 = local write "Pause Data Collection"(TRUE ("Pause Data Collection")) -> ()
                                n4906 = Wait (ms)(milliseconds to wait=u32 500) -> ()  [unwired: 1 out]
                                n4907 = call "PortChanger (SubVI).vi"("Port Number"=w5331, "VISA Refnum in"=w5332) -> ()  [unwired: 10 in]
                                }
                                frame #8 {
                                n4908 = local read "VISA Refnum in\nfor Pump"() -> (w5335:refnum<visa-resource-name>)
                                n4909 = local write "Volume being Injected \nin this process"(0.0 ("Volume being Injected \nin this process")) -> ()
                                n4910 = call "ProcessCompletionWaiter (SubVI).vi"("VISA Refnum in"=w5335) -> ()  [unwired: 11 in]
                                }
                              }
                            }
                            n4911 = local write "Reminder of the \nVolume to be \nPumped"(w5266) -> ()
                          }
                          frame #4 {
                            n4912 = stacked-sequence {
                              frame #0 {
                                n4913 = local read "Buffer-A2 PickUp \nFlow Rate (ul/min)"() -> (w5339:dbl)
                                n4914 = local read "Buffer-A2 Pumping\nResolution"() -> (w5338:T2)
                                n4915 = local read "VISA Refnum in\nfor Pump"() -> (w5341:refnum<visa-resource-name>)
                                n4916 = local read "Reminder of the \nVolume to be \nPumped"() -> (w5337:dbl)
                                n4917 = local read "Volume of Syringe"() -> (w5340:dbl)
                                n4918 = call "RPickUp(SubVI).vi"("Volume to be picked up"=w5337, "Volume of Syringe"=w5340, "Resolution of PickUP"=w5338, "PickUp Flow Rate (ul/min)"=w5339, "VISA Refnum in"=w5341) -> ()  [unwired: 6 in, 1 out]
                              }
                              frame #1 {
                                n4919 = local read "Stopper that ends \nthe main loops"() -> (w5342:bool)
                                n4920 = local read "VISA Refnum in\nfor Pump"() -> (w5343:refnum<visa-resource-name>)
                                n4921 = case shown="True" w5342 {
                                frame False {
                                }
                                frame True {
                                n4922 = local read "VISA Refnum in\nfor Pump"() -> (w5344:refnum<visa-resource-name>)
                                n4923 = call "HardStopCurrentProcess (SubVI).vi"("VISA Refnum in"=w5344) -> ()  [unwired: 11 in]
                                }
                                }
                                n4924 = call "ProcessCompletionWaiter (SubVI).vi"("VISA Refnum in"=w5343) -> ()  [unwired: 11 in]
                              }
                              frame #2 {
                                # "Reads the initial Plunger Position for computing the volume dispensed"
                                n4925 = local read "VISA Refnum in\nfor Pump"() -> (w5346:refnum<visa-resource-name>)
                                n4926 = call "AbsolutePlungerPosition (SubVI).vi"("VISA Refnum in"=w5346) -> ("Plunger Position"=w5345:i32)  [unwired: 10 in]
                                n4927 = local write "Initial Plunger Position"(w5345) -> ()
                              }
                              frame #3 {
                                # "Switch to Port-2"
                                # "Port-2 of the pump is conncted to column-1 of chip"
                                n4928 = local read "VISA Refnum in\nfor Pump"() -> (w5348:refnum<visa-resource-name>)
                                n4929 = call "PortChanger (SubVI).vi"("Port Number"="2", "VISA Refnum in"=w5348) -> ()  [unwired: 10 in]
                              }
                              frame #4 {
                                n4930 = local read "Stopper that ends \nthe main loops"() -> (w5349:bool)
                                n4931 = local read "VISA Refnum in\nfor Pump"() -> (w5350:refnum<visa-resource-name>)
                                n4932 = case shown="True" w5349 {
                                frame False {
                                }
                                frame True {
                                n4933 = local read "VISA Refnum in\nfor Pump"() -> (w5351:refnum<visa-resource-name>)
                                n4934 = call "HardStopCurrentProcess (SubVI).vi"("VISA Refnum in"=w5351) -> ()  [unwired: 11 in]
                                }
                                }
                                n4935 = call "ProcessCompletionWaiter (SubVI).vi"("VISA Refnum in"=w5350) -> ()  [unwired: 11 in]
                              }
                              frame #5 {
                                # "Keeps the AMF valve after column-1 open and valve after column-2 closed"
                                n4936 = local read "Buffer-A2 Dispense\nFlow Rate (ul/min)"() -> (w5355:dbl)
                                n4937 = local read "Buffer-A2 Pumping\nResolution"() -> (w5354:T2)
                                n4938 = local read "VISA Refnum in\nfor Pump"() -> (w5357:refnum<visa-resource-name>)
                                n4939 = local write "Pause Data Collection"(FALSE ("Pause Data Collection")) -> ()
                                n4940 = local read "Volume of Syringe"() -> (w5356:dbl)
                                n4941 = call "GoToAbsolutePosition(SubVI).vi"("Absolute Volume Position in Syringe (in ul)"=0.0 ("Volume to be Dispensed"), "Volume of Syringe"=w5356, "Resolution of Pumping"=w5354, "Flow Rate (ul/min)"=w5355, "VISA Refnum in"=w5357) -> ()  [unwired: 6 in, 1 out]
                              }
                              frame #6 {
                                n4942 = local read "Buffer-A2 Pumping\nResolution"() -> (w5359:T2)
                                n4943 = local read "VISA Refnum in\nfor Pump"() -> (w5361:refnum<visa-resource-name>)
                                n4944 = local read "Initial Plunger Position"() -> (w5360:dbl)
                                n4945 = local read "Volume of Syringe"() -> (w5358:dbl)
                                n4946 = while {
                                tunnel: w5360 -> [w5368]
                                tunnel: w5361 -> [w5367]
                                tunnel: w5359 -> [w5366]
                                tunnel: w5358 -> [w5365]
                                stop <- w5363 stop-if-true
                                n4947 = stacked-sequence {
                                tunnel: w5368 -> [w5375 _]
                                tunnel: w5367 -> [w5374 w5395]
                                tunnel: w5366 -> [w5373 _]
                                tunnel: w5365 -> [w5372 _]
                                tunnel: [_ w5393] -> w5363
                                frame #0 {
                                n4948 = call "AbsolutePlungerPosition (SubVI).vi"("VISA Refnum in"=w5374) -> ("Plunger Position"=w5371:i32)  [unwired: 10 in]
                                n4949 = case shown="\"Standard Pumping\", Default" w5373 {
                                tunnel: w5375 -> [w5380 w5389]
                                tunnel: w5371 -> [w5381 w5388]
                                tunnel: [w5379 w5386] -> w5370
                                tunnel: w5372 -> [w5378 w5387]
                                frame "Standard Pumping", Default {
                                n4950 = Subtract(x=w5380, y=w5381) -> (x-y=w5377:dbl)
                                n4951 = Absolute Value(x=w5377) -> (abs(x)=w5376:dbl)
                                n4952 = Multiply(x=w5376, y=w5378) -> (x*y=w5383:dbl)
                                n4953 = Divide(x=w5383, y=3000.0) -> (x/y=w5379:dbl)
                                }
                                frame "High Resolution Pumping" {
                                n4954 = Subtract(x=w5389, y=w5388) -> (x-y=w5385:dbl)
                                n4955 = Absolute Value(x=w5385) -> (abs(x)=w5384:dbl)
                                n4956 = Multiply(x=w5384, y=w5387) -> (x*y=w5391:dbl)
                                n4957 = Divide(x=w5391, y=24000.0) -> (x/y=w5386:dbl)
                                }
                                }
                                n4958 = local write "Volume being Injected \nin this process"(w5370) -> ()
                                }
                                frame #1 {
                                n4959 = call "LSPOneStatus (SubVI).vi"("VISA Refnum in"=w5395) -> ("read buffer"=w5397:string)  [unwired: 10 in]
                                n4960 = call <vilib>:"Trim Whitespace.vi"("string"=w5397) -> ("trimmed string"=w5396:string)  [unwired: 1 in]
                                n4961 = local read "Stopper that ends \nthe main loops"() -> (w5392:bool)
                                n4962 = Equal?(x=w5396, y="/0`\u0003") -> (x = y?=w5394:bool)
                                n4963 = Or(x=w5394, y=w5392) -> (x .or. y?=w5393:bool)
                                }
                                }
                                n4964 = Wait (ms)(milliseconds to wait=u32 100) -> ()  [unwired: 1 out]
                                n4965 = local read "Stopper that ends \nthe main loops"() -> (w5362:bool)
                                n4966 = case shown="True" w5362 {
                                frame False {
                                }
                                frame True {
                                n4967 = local read "VISA Refnum in\nfor Pump"() -> (w5369:refnum<visa-resource-name>)
                                n4968 = call "HardStopCurrentProcess (SubVI).vi"("VISA Refnum in"=w5369) -> ()  [unwired: 11 in]
                                }
                                }
                                }
                              }
                              frame #7 {
                                n4969 = local write "Pause Data Collection"(TRUE ("Pause Data Collection")) -> ()
                                n4970 = Wait (ms)(milliseconds to wait=u32 500) -> ()  [unwired: 1 out]
                              }
                              frame #8 {
                                n4971 = local write "Volume being Injected \nin this process"(0.0 ("Volume being Injected \nin this process")) -> ()
                                n4972 = local write "Start the Process"(FALSE ("Start the Process")) -> ()
                              }
                            }
                          }
                        }
                        n4973 = local write "Washing Column-1"(TRUE ("Washing Column-1")) -> ()
                      }
                      frame #3 {
                        # "Connecting Buffer-C with port-5, cleaning the tubing with Buffer-C1, and washing the Column-2 to get rid of spill out from wash steps of column-1"
                        n4974 = local write "Washing Column-1"(FALSE ("Washing Column-1")) -> ()
                        n4975 = stacked-sequence {
                          frame #0 {
                            # "Switch to Port-5"
                            # "Port-5 of pump is connected to Buffer-C1"
                            n4976 = local read "VISA Refnum in\nfor Pump"() -> (w5406:refnum<visa-resource-name>)
                            n4977 = local read "Port for \nC1-Equilibriation"() -> (w5405:string)
                            n4978 = call "PortChanger (SubVI).vi"("Port Number"=w5405, "VISA Refnum in"=w5406) -> ()  [unwired: 10 in]
                          }
                          frame #1 {
                            n4979 = local read "VISA Refnum in\nfor Pump"() -> (w5407:refnum<visa-resource-name>)
                            n4980 = call "ProcessCompletionWaiter (SubVI).vi"("VISA Refnum in"=w5407) -> ()  [unwired: 11 in]
                          }
                          frame #2 {
                            # "Wash the inside of the pump valve"
                            n4981 = local read "n"() -> (w5408:i32)
                            n4982 = for {
                              N: w5408 -> [_]
                              n4983 = stacked-sequence {
                                frame #0 {
                                n4984 = local read "Buffer-A2 Pumping\nResolution"() -> (w5411:T2)
                                n4985 = local read "VISA Refnum in\nfor Pump"() -> (w5413:refnum<visa-resource-name>)
                                n4986 = local read "V-S"() -> (w5409:dbl)
                                n4987 = local read "Volume of Syringe"() -> (w5412:dbl)
                                n4988 = call "RPickUp(SubVI).vi"("Volume to be picked up"=w5409, "Volume of Syringe"=w5412, "Resolution of PickUP"=w5411, "PickUp Flow Rate (ul/min)"=150.0, "VISA Refnum in"=w5413) -> ()  [unwired: 6 in, 1 out]
                                }
                                frame #1 {
                                n4989 = local read "Stopper that ends \nthe main loops"() -> (w5414:bool)
                                n4990 = local read "VISA Refnum in\nfor Pump"() -> (w5415:refnum<visa-resource-name>)
                                n4991 = case shown="True" w5414 {
                                frame False {
                                }
                                frame True {
                                n4992 = local read "VISA Refnum in\nfor Pump"() -> (w5416:refnum<visa-resource-name>)
                                n4993 = call "HardStopCurrentProcess (SubVI).vi"("VISA Refnum in"=w5416) -> ()  [unwired: 11 in]
                                }
                                }
                                n4994 = call "ProcessCompletionWaiter (SubVI).vi"("VISA Refnum in"=w5415) -> ()  [unwired: 11 in]
                                }
                                frame #2 {
                                # "Switch to Port-1"
                                # "Port-1 of the pump is conncted to waste"
                                n4995 = local read "VISA Refnum in\nfor Pump"() -> (w5418:refnum<visa-resource-name>)
                                n4996 = call "PortChanger (SubVI).vi"("Port Number"="1", "VISA Refnum in"=w5418) -> ()  [unwired: 10 in]
                                }
                                frame #3 {
                                n4997 = local read "Stopper that ends \nthe main loops"() -> (w5419:bool)
                                n4998 = local read "VISA Refnum in\nfor Pump"() -> (w5420:refnum<visa-resource-name>)
                                n4999 = case shown="True" w5419 {
                                frame False {
                                }
                                frame True {
                                n5000 = local read "VISA Refnum in\nfor Pump"() -> (w5421:refnum<visa-resource-name>)
                                n5001 = call "HardStopCurrentProcess (SubVI).vi"("VISA Refnum in"=w5421) -> ()  [unwired: 11 in]
                                }
                                }
                                n5002 = call "ProcessCompletionWaiter (SubVI).vi"("VISA Refnum in"=w5420) -> ()  [unwired: 11 in]
                                }
                                frame #4 {
                                n5003 = local read "Buffer-A2 Pumping\nResolution"() -> (w5424:T2)
                                n5004 = local read "VISA Refnum in\nfor Pump"() -> (w5426:refnum<visa-resource-name>)
                                n5005 = local read "Volume of Syringe"() -> (w5425:dbl)
                                n5006 = call "GoToAbsolutePosition(SubVI).vi"("Absolute Volume Position in Syringe (in ul)"=0.0 ("Volume to be Dispensed"), "Volume of Syringe"=w5425, "Resolution of Pumping"=w5424, "Flow Rate (ul/min)"=150.0, "VISA Refnum in"=w5426) -> ()  [unwired: 6 in, 1 out]
                                }
                                frame #5 {
                                n5007 = local read "VISA Refnum in\nfor Pump"() -> (w5427:refnum<visa-resource-name>)
                                n5008 = call "ProcessCompletionWaiter (SubVI).vi"("VISA Refnum in"=w5427) -> ()  [unwired: 11 in]
                                }
                                frame #6 {
                                # "Change the port back to Buffer-C1"
                                n5009 = local read "VISA Refnum in\nfor Pump"() -> (w5429:refnum<visa-resource-name>)
                                n5010 = local read "Port for \nC1-Equilibriation"() -> (w5428:string)
                                n5011 = call "PortChanger (SubVI).vi"("Port Number"=w5428, "VISA Refnum in"=w5429) -> ()  [unwired: 10 in]
                                }
                                frame #7 {
                                n5012 = local read "VISA Refnum in\nfor Pump"() -> (w5430:refnum<visa-resource-name>)
                                n5013 = call "ProcessCompletionWaiter (SubVI).vi"("VISA Refnum in"=w5430) -> ()  [unwired: 11 in]
                                }
                              }
                            }
                          }
                          frame #3 {
                            # "Wash the pathway between column-2 and column-1 on chip"
                            n5014 = local read "n"() -> (w5431:i32)
                            n5015 = for {
                              N: w5431 -> [_]
                              n5016 = stacked-sequence {
                                frame #0 {
                                n5017 = local read "Buffer-A2 Pumping\nResolution"() -> (w5434:T2)
                                n5018 = local read "VISA Refnum in\nfor Pump"() -> (w5436:refnum<visa-resource-name>)
                                n5019 = local read "V-S"() -> (w5432:dbl)
                                n5020 = local read "Volume of Syringe"() -> (w5435:dbl)
                                n5021 = call "RPickUp(SubVI).vi"("Volume to be picked up"=w5432, "Volume of Syringe"=w5435, "Resolution of PickUP"=w5434, "PickUp Flow Rate (ul/min)"=150.0, "VISA Refnum in"=w5436) -> ()  [unwired: 6 in, 1 out]
                                }
                                frame #1 {
                                n5022 = local read "Stopper that ends \nthe main loops"() -> (w5437:bool)
                                n5023 = local read "VISA Refnum in\nfor Pump"() -> (w5438:refnum<visa-resource-name>)
                                n5024 = case shown="True" w5437 {
                                frame False {
                                }
                                frame True {
                                n5025 = local read "VISA Refnum in\nfor Pump"() -> (w5439:refnum<visa-resource-name>)
                                n5026 = call "HardStopCurrentProcess (SubVI).vi"("VISA Refnum in"=w5439) -> ()  [unwired: 11 in]
                                }
                                }
                                n5027 = call "ProcessCompletionWaiter (SubVI).vi"("VISA Refnum in"=w5438) -> ()  [unwired: 11 in]
                                }
                                frame #2 {
                                # "Switch to Port-10"
                                # "Port-10 of the pump is conncted to column-2"
                                n5028 = local read "VISA Refnum in\nfor Pump"() -> (w5441:refnum<visa-resource-name>)
                                n5029 = call "PortChanger (SubVI).vi"("Port Number"="10", "VISA Refnum in"=w5441) -> ()  [unwired: 10 in]
                                }
                                frame #3 {
                                n5030 = local read "Stopper that ends \nthe main loops"() -> (w5442:bool)
                                n5031 = local read "VISA Refnum in\nfor Pump"() -> (w5443:refnum<visa-resource-name>)
                                n5032 = case shown="True" w5442 {
                                frame False {
                                }
                                frame True {
                                n5033 = local read "VISA Refnum in\nfor Pump"() -> (w5444:refnum<visa-resource-name>)
                                n5034 = call "HardStopCurrentProcess (SubVI).vi"("VISA Refnum in"=w5444) -> ()  [unwired: 11 in]
                                }
                                }
                                n5035 = call "ProcessCompletionWaiter (SubVI).vi"("VISA Refnum in"=w5443) -> ()  [unwired: 11 in]
                                }
                                frame #4 {
                                n5036 = local read "Buffer-A2 Pumping\nResolution"() -> (w5452:T2)
                                n5037 = local read "VISA Refnum in\nfor Pump"() -> (w5454:refnum<visa-resource-name>)
                                n5038 = local read "f"() -> (w5446:dbl)
                                n5039 = local read "Volume of Syringe"() -> (w5453:dbl)
                                n5040 = call "GoToAbsolutePosition(SubVI).vi"("Absolute Volume Position in Syringe (in ul)"=0.0 ("Volume to be Dispensed"), "Volume of Syringe"=w5453, "Resolution of Pumping"=w5452, "Flow Rate (ul/min)"=w5446, "VISA Refnum in"=w5454) -> ()  [unwired: 6 in, 1 out]
                                n5041 = local write "External Valve \nOpen"(TRUE ("External Valve \nOpen")) -> ()
                                n5042 = local write "Valve V2 Open"(TRUE ("Valve V2 Open")) -> ()
                                n5043 = local write "Valve V1 Open"(FALSE ("Valve V1 Open")) -> ()
                                n5044 = local write "Valve V4 Open"(FALSE ("Valve V4 Open")) -> ()
                                n5045 = local write "Valve V3 Open"(TRUE ("Valve V3 Open")) -> ()
                                }
                                frame #5 {
                                n5046 = local read "VISA Refnum in\nfor Pump"() -> (w5455:refnum<visa-resource-name>)
                                n5047 = call "ProcessCompletionWaiter (SubVI).vi"("VISA Refnum in"=w5455) -> ()  [unwired: 11 in]
                                }
                                frame #6 {
                                # "Change the port back to Buffer-C1"
                                n5048 = local read "VISA Refnum in\nfor Pump"() -> (w5457:refnum<visa-resource-name>)
                                n5049 = local read "Port for \nC1-Equilibriation"() -> (w5456:string)
                                n5050 = call "PortChanger (SubVI).vi"("Port Number"=w5456, "VISA Refnum in"=w5457) -> ()  [unwired: 10 in]
                                }
                                frame #7 {
                                n5051 = local read "VISA Refnum in\nfor Pump"() -> (w5458:refnum<visa-resource-name>)
                                n5052 = call "ProcessCompletionWaiter (SubVI).vi"("VISA Refnum in"=w5458) -> ()  [unwired: 11 in]
                                }
                              }
                            }
                          }
                          frame #4 {
                            # "Washes the SEC column"
                            n5053 = local read "Apparent Volume\nof Syringe"() -> (w5461:dbl)
                            n5054 = local read "c"() -> (w5462:dbl)
                            n5055 = Quotient & Remainder(x=w5462, y=w5461) -> (x-y*floor(x/y)=w5460:dbl, floor(x/y)=w5459:dbl)
                            n5056 = for {
                              N: w5459 -> [_]
                              n5057 = stacked-sequence {
                                frame #0 {
                                n5058 = local read "Buffer-A2 Pumping\nResolution"() -> (w5465:T2)
                                n5059 = local read "VISA Refnum in\nfor Pump"() -> (w5467:refnum<visa-resource-name>)
                                n5060 = local read "Apparent Volume\nof Syringe"() -> (w5463:dbl)
                                n5061 = local read "Volume of Syringe"() -> (w5466:dbl)
                                n5062 = call "RPickUp(SubVI).vi"("Volume to be picked up"=w5463, "Volume of Syringe"=w5466, "Resolution of PickUP"=w5465, "PickUp Flow Rate (ul/min)"=150.0, "VISA Refnum in"=w5467) -> ()  [unwired: 6 in, 1 out]
                                }
                                frame #1 {
                                n5063 = local read "Stopper that ends \nthe main loops"() -> (w5468:bool)
                                n5064 = local read "VISA Refnum in\nfor Pump"() -> (w5469:refnum<visa-resource-name>)
                                n5065 = case shown="True" w5468 {
                                frame False {
                                }
                                frame True {
                                n5066 = local read "VISA Refnum in\nfor Pump"() -> (w5470:refnum<visa-resource-name>)
                                n5067 = call "HardStopCurrentProcess (SubVI).vi"("VISA Refnum in"=w5470) -> ()  [unwired: 11 in]
                                }
                                }
